vi "Create.vi"(7 "Core User Interfaces":refnum<class "Core User Interfaces.lvclass">, 8 "error in (no error)":errorcluster, 9 "user interface type":T1, 10 "component settings":T2[](array[typedef]), 11 "Components":refnum<class "Component.lvclass">[](array[class])) -> (0 "error out":errorcluster, 3 "Settings Editor out":refnum<class "Settings Editor.lvclass">)   [LabVIEW 2017, in "DSF Core.lvlib" / "Settings Editor.lvclass"]
uses:
  Settings Editor.lvclass
  Component/Component.lvclass
  Typedefs/DSF Settings Info.ctl
  Typedefs/DSF Version Info.ctl
  Component User Interface/UI Type.ctl
  Core/Core User Interfaces.lvclass
  C:/Git/DSF/Core/Classes/Component User Interface/Component User Interfaces.lvclass
  Settings Editor.lvclass/Settings Editor.ctl
  Plugin/Component Settings Editor.lvclass
  Component User Interface/Component User Interfaces.lvclass
  DSF Core.lvlib
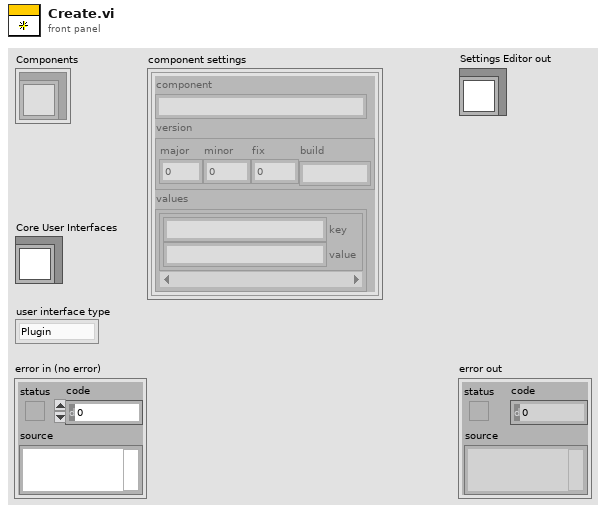
[diagram p1: front panel]
types:
  T1 = typedef "DSF Core.lvlib/Component User Interfaces.lvclass/UI Type.ctl" = enum16{"Plugin", "Thread", "Rx Group", "Tx Group", "Rx Transfer", "Tx Transfer", "Rx Channel", "Tx Channel"}
  T2 = typedef "DSF Core.lvlib/DSF Settings Info.ctl" = cluster{"component":string, "version":T3, "values":cluster{"key":string, "value":string}[]}
  T3 = typedef "DSF Core.lvlib/DSF Version Info.ctl" = cluster{"major":u32, "minor":u32, "fix":u32, "build":string}
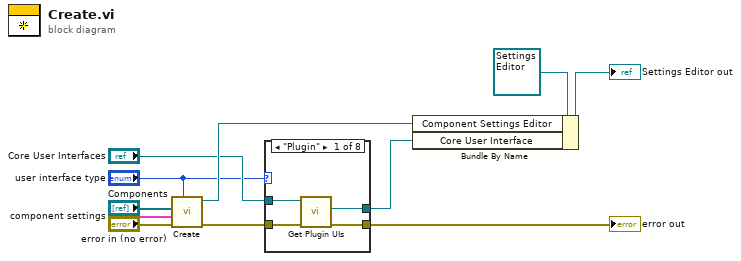
[diagram p0: block diagram]
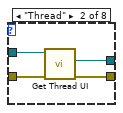
[diagram p2: hidden frame]
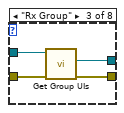
[diagram p3: hidden frame]
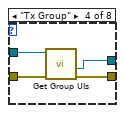
[diagram p4: hidden frame]
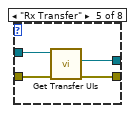
[diagram p5: hidden frame]
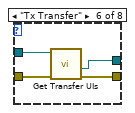
[diagram p6: hidden frame]
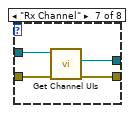
[diagram p7: hidden frame]
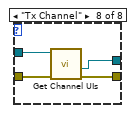
[diagram p8: hidden frame]
diagram:
  n1 = call "Create.vi"("user interface type"="user interface type", "error in (no error)"="error in (no error)", "component settings"="component settings", "Components"="Components") -> ("error out"=w4:errorcluster, "Component Settings Editor out"=w7:refnum<class "Component Settings Editor.lvclass">)  [unwired: 6 in]
  n2 = case shown="\"Plugin\"" "user interface type" {
    tunnel: [w15 w19 w23 w26 w31 w34 w36 w40] -> w1
    tunnel: "Core User Interfaces" -> [w14 w18 w22 w27 w30 w35 w39 w43]
    tunnel: [w12 w16 w20 w24 w28 w32 w37 w41] -> w3
    tunnel: w4 -> [w13 w17 w21 w25 w29 w33 w38 w42]
    frame "Plugin" {
      n3 = call "Get Plugin UIs.vi"("error in (no error)"=w13, "Component UI in"=w14) -> ("error out"=w12:errorcluster, "Plugin Settings UI"=w15:refnum<class "User Interface.lvclass">)  [unwired: 7 in, 1 out]
    }
    frame "Thread" {
      n4 = call "Get Thread UI.vi"("error in (no error)"=w17, "Component UI in"=w18) -> ("error out"=w16:errorcluster, "Thread Settings UI"=w19:refnum<class "User Interface.lvclass">)  [unwired: 7 in, 1 out]
    }
    frame "Rx Group" {
      n5 = call "Get Group UIs.vi"("error in (no error)"=w21, "Component UI in"=w22) -> ("error out"=w20:errorcluster, "Rx Group UI"=w23:refnum<class "User Interface.lvclass">)  [unwired: 6 in, 2 out]
    }
    frame "Tx Group" {
      n6 = call "Get Group UIs.vi"("error in (no error)"=w25, "Component UI in"=w27) -> ("error out"=w24:errorcluster, "Tx Group UI"=w26:refnum<class "User Interface.lvclass">)  [unwired: 6 in, 2 out]
    }
    frame "Rx Transfer" {
      n7 = call "Get Transfer UIs.vi"("error in (no error)"=w29, "Component UI in"=w30) -> ("error out"=w28:errorcluster, "Rx Transfer UI"=w31:refnum<class "User Interface.lvclass">)  [unwired: 6 in, 2 out]
    }
    frame "Tx Transfer" {
      n8 = call "Get Transfer UIs.vi"("error in (no error)"=w33, "Component UI in"=w35) -> ("error out"=w32:errorcluster, "Tx Transfer UI"=w34:refnum<class "User Interface.lvclass">)  [unwired: 6 in, 2 out]
    }
    frame "Rx Channel" {
      n9 = call "Get Channel UIs.vi"("error in (no error)"=w38, "Component UI in"=w39) -> ("error out"=w37:errorcluster, "Rx Channel UI"=w36:refnum<class "User Interface.lvclass">)  [unwired: 6 in, 2 out]
    }
    frame "Tx Channel" {
      n10 = call "Get Channel UIs.vi"("error in (no error)"=w42, "Component UI in"=w43) -> ("error out"=w41:errorcluster, "Tx Channel UI"=w40:refnum<class "User Interface.lvclass">)  [unwired: 6 in, 2 out]
    }
  }
  "error out" <- w3
  n11 = Bundle By Name(cluster=refnum<class "Settings Editor.lvclass"> refnum ("Settings Editor in"), "Component Settings Editor"=w7, "Core User Interface"=w1) -> (→"Settings Editor out":refnum<class "Settings Editor.lvclass">)
